vi "Test MQTT-1.5.3-2.vi"(8 "error in (no error)":errorcluster) -> (0 "error out":errorcluster)   [LabVIEW 2013]
uses:
  <vilib>/addons/_JKI Toolkits/Caraya/classes/Test/Test.lvclass
  source/Control Packets/ControlPacket/ControlPacket.lvclass
  <vilib>/addons/_JKI Toolkits/Caraya/classes/Assert/Assert.lvclass
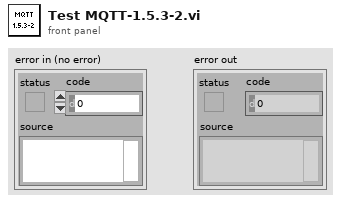
[diagram p1: front panel]
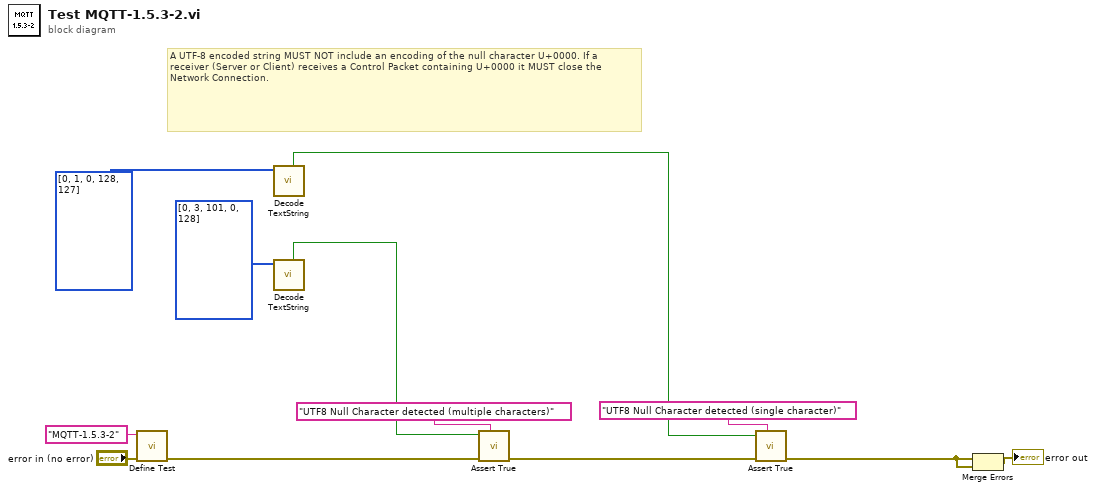
[diagram p0: block diagram]
diagram:
  # "A UTF-8 encoded string MUST NOT include an encoding of the null character U+0000. If a receiver (Server or Client) receives a Control Packet containing U+0000 it MUST close the Network Connection."
  n1 = call <vilib>:"Define Test.vi"("error in (no error)"="error in (no error)", "Label (VI Title)"="MQTT-1.5.3-2") -> ("error out"=w1:errorcluster)  [unwired: 9 in]
  n2 = call "Decode TextString.vi"("Length-Prefixed Field"=u8[] [0, 1, 0, 128, 127]) -> ("restricted code"=w2:bool)  [unwired: 8 in, 2 out]
  n3 = call "Decode TextString.vi"("Length-Prefixed Field"=u8[] [0, 3, 101, 0, 128]) -> ("restricted code"=w7:bool)  [unwired: 8 in, 2 out]
  n4 = call <vilib>:"Assert True.vi"("Label"="UTF8 Null Character detected (multiple characters)", "error in (no error)"=w1, "True?"=w7) -> ("error out"=w4:errorcluster)  [unwired: 8 in]
  n5 = call <vilib>:"Assert True.vi"("Label"="UTF8 Null Character detected (single character)", "error in (no error)"=w4, "True?"=w2) -> ("error out"=w3:errorcluster)  [unwired: 8 in]
  n6 = Merge Errors(w3, w3) -> (→"error out":errorcluster)
